vi "PacketSplitter.vi"(3 "Ratio":dbl[](array[numeric]), 4 "Channel Array In":T1(array[cluster])) -> (1 "Remained\nData":u8[](array[numeric]))   [LabVIEW 2014]
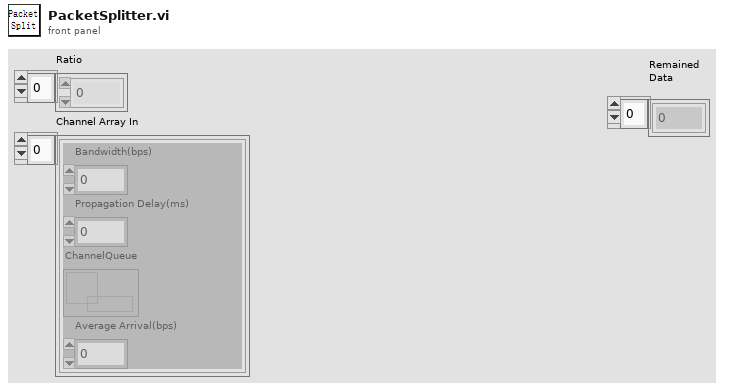
[diagram p1: front panel]
types:
  T1 = cluster{"Bandwidth(bps)":i32, "Propagation Delay(ms)":i32, "ChannelQueue":refnum<queue>, "Average Arrival(bps)":dbl}[]
  T2 = cluster{"Sequence":i32, "Data":u8[], "Timestamp":i32}
  T3 = cluster{"Sequence":i32, "Data":u8[], "PacketSize":i32, "Offset":i32, "FragmentSize":i32, "Timestamp":i32}
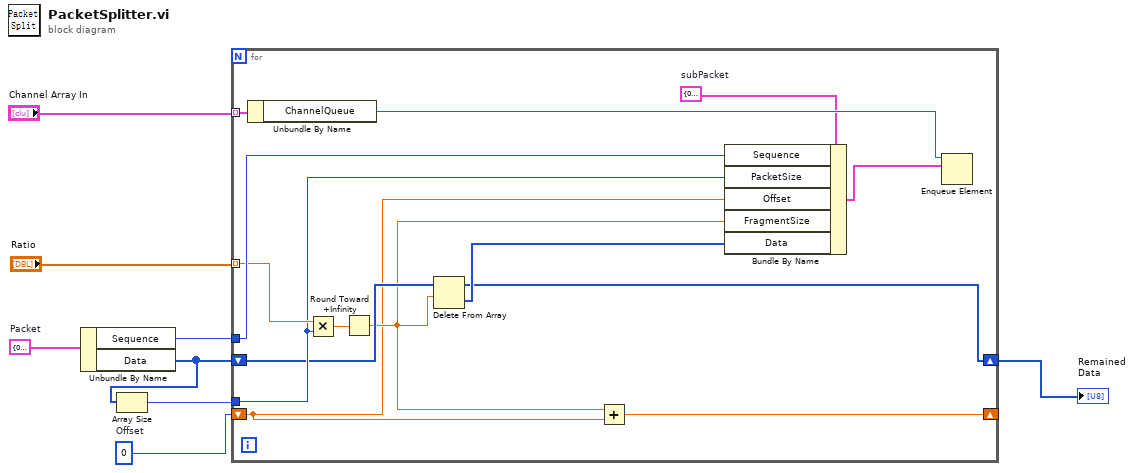
[diagram p0: block diagram]
diagram:
  w1 = T2 {"Sequence"=0, "Data"=[], "Timestamp"=0}  # Packet
  w3 = 0  # Offset
  n1 = Unbundle By Name(w1) -> ("Sequence"=w6:i32, "Data"=w5:u8[])
  n2 = Array Size(array=w5) -> (size(s)=w4:i32)
  n3 = for {
    tunnel: "Channel Array In" -> [w21] mode=indexing
    tunnel: "Ratio" -> [w18] mode=indexing
    tunnel: w6 -> [w22]
    shift-right: [w13] -> w2
    shift-left: w5 -> [w15]
    tunnel: w4 -> [w17]
    shift-right: [w11] -> _
    shift-left: w3 -> [w10]
    w9 = T3 {"Sequence"=0, "Data"=[], "PacketSize"=0, "Offset"=0, "FragmentSize"=0, "Timestamp"=0}  # subPacket
    n4 = Unbundle By Name(w21) -> ("ChannelQueue"=w20:refnum<queue>)
    n5 = Multiply(x=w18, y=w17) -> (x*y=w16:dbl)
    n6 = Round Toward +Infinity(x=w16) -> (ceil(x): smallest int >= x=w12:dbl)
    n7 = Delete From Array(array=w15, length=w12) -> (deleted portion=w14:u8[], array with subset deleted=w13:u8[])  [unwired: 1 in]
    n8 = Add(x=w12, y=w10) -> (x+y=w11:dbl)
    n9 = Bundle By Name(cluster=w9, "Sequence"=w22, "PacketSize"=w17, "Offset"=w10, "FragmentSize"=w12, "Data"=w14) -> (w19:T3)
    n10 = Enqueue Element(queue=w20, element=w19) -> ()  [unwired: 2 in, 3 out]
  }
  "Remained\nData" <- w2
